vi "Configure Edge Trigger.vi"(0 "VISA resource name":refnum<visa-resource-name>, 1 "Trigger Slope (0: Rising)":u16(ring) items=["Rising", "Falling"], 2 "Trigger Source (0: Channel 1)":u16(ring) items=["Channel 1", "Channel 2", "Channel 3", "Channel 4", "External", "Line", "Ext", "Ext10"], 5 "Trigger Level (0.0 V)":dbl, 9 "Holdoff Type (0: Time)":u16(ring) items=["Time", "Events", "None"], 11 "error in (no error)":errorcluster, 12 "Holdoff Value by Time (50 ns)":dbl=5e-08, 14 "Holdoff Value by Events (1)":i32=1) -> (4 "VISA resource name out":refnum<visa-resource-name>, 15 "error out":errorcluster)   [LabVIEW 2013, in "LeCroy Wave Series.lvlib"]
doc: "Configures edge trigger settings. An edge trigger occurs when the trigger signal passes through the voltage threshold that you specify with the Level control and has the slope that you specify with the Slope control. \n\nNote: \"External\" is included for the purpose of backwards compatibility. Use EXT or EXT10 for best results."
uses:
  LeCroy Wave Series.lvlib
panel:
  # "Note: \"External\" is included for the purpose\nof backwards compatibility.  Use EXT or EXT10\nfor best results."
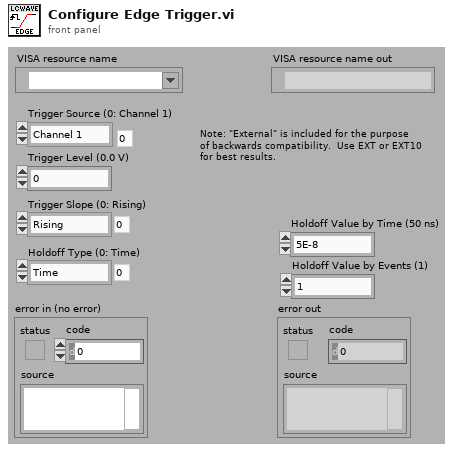
[diagram p1: front panel]
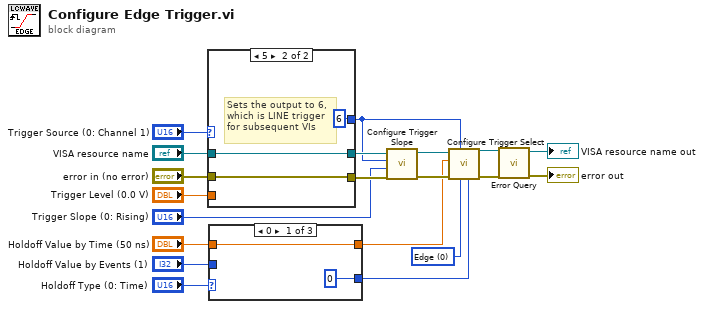
[diagram p0: block diagram]
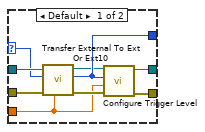
[diagram p2: hidden frame]
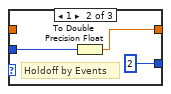
[diagram p3: hidden frame]
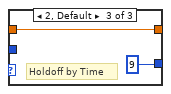
[diagram p4: hidden frame]
diagram:
  w2 = u16 0 items=["Edge", "Dropout", "Glitch", "Interval", "Std", "Sng", "State Qualify", "Edge Qualify"] ("Trigger type")
  n1 = case shown="5" "Trigger Source (0: Channel 1)" {
    selector: "Trigger Source (0: Channel 1)" -> [w22 _]
    tunnel: "Trigger Level (0.0 V)" -> [w21 _]
    tunnel: [w29 w32] -> w19
    tunnel: [w28 w31] -> w18
    tunnel: "VISA resource name" -> [w24 w32]
    tunnel: "error in (no error)" -> [w26 w31]
    tunnel: [w27 6] -> w4
    frame Default {
      n2 = call "Transfer External To Ext Or Ext10.vi"("Trigger Level"=w21, "error in (no error)"=w26, "Trigger Source With External"=w22, "VISA resource name"=w24) -> ("error out"=w25:errorcluster, "Trigger Source With Ext/Ext10"=w27:u16, "VISA resource name out"=w23:refnum<visa-resource-name>)  [unwired: 5 in]
      n3 = call "Configure Trigger Level.vi"("error in (no error)"=w25, "Trigger Level 1 (0.0 V)"=w21, "Channel (0: Channel 1)"=w27, "VISA resource name"=w23) -> ("error out"=w28:errorcluster, "VISA resource name out"=w29:refnum<visa-resource-name>)  [unwired: 6 in]
    }
    frame 5 {
      # "Sets the output to 6,\nwhich is LINE trigger\nfor subsequent VIs"
    }
  }
  n4 = case shown="0" "Holdoff Type (0: Time)" {
    tunnel: [w34 w35 w39] -> w3
    tunnel: "Holdoff Value by Time (50 ns)" -> [w34 _ w39]
    tunnel: "Holdoff Value by Events (1)" -> [_ w36 _]
    tunnel: [0 2 9] -> w1
    frame 0 {
    }
    frame 1 {
      # "Holdoff by Events"
      n5 = To Double Precision Float(number=w36) -> (double precision float=w35:dbl)
    }
    frame 2, Default {
      # "Holdoff by Time"
    }
  }
  n6 = call "Configure Trigger Slope.vi"("error in (no error)"=w18, "Trigger Slope (0: Rising)"="Trigger Slope (0: Rising)", "Channel (0: Channel 1)"=w4, "VISA resource name"=w19) -> ("error out"=w15:errorcluster, "VISA resource name out"=w16:refnum<visa-resource-name>)  [unwired: 6 in]
  n7 = call "Configure Trigger Select.vi"("Hold Type (0: TI)"=w1, "Trigger type"=w2, "Trigger Source (0: Channel 1)"=w4, "error in (no error)"=w15, "Hold Value 1 (4 ns)"=w3, "VISA resource name"=w16) -> ("error out"=w6:errorcluster, "VISA resource name out"=w7:refnum<visa-resource-name>)  [unwired: 4 in]
  n8 = call "Error Query.vi"("error in (no error)"=w6, "VISA resource name"=w7) -> ("error out"=→"error out":errorcluster, "VISA resource name out"=→"VISA resource name out":refnum<visa-resource-name>)  [unwired: 6 in, 2 out]
